vi "Get eq of Time.vi"(6 "Eccentricity":dbl, 9 "Mean Anomaly":dbl, 10 "Geometric Mean Longitude":dbl, 11 "Oblique Correction (deg)":dbl) -> (2 "Eq of Time (min)":dbl, 3 "var y":dbl)   [LabVIEW 2014, in "Solar Calculations.lvlib"]
uses:
  Solar Calculations.lvlib
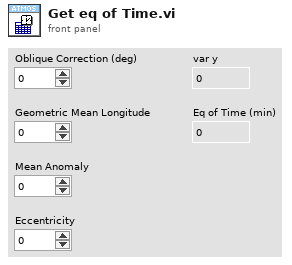
[diagram p1: front panel]
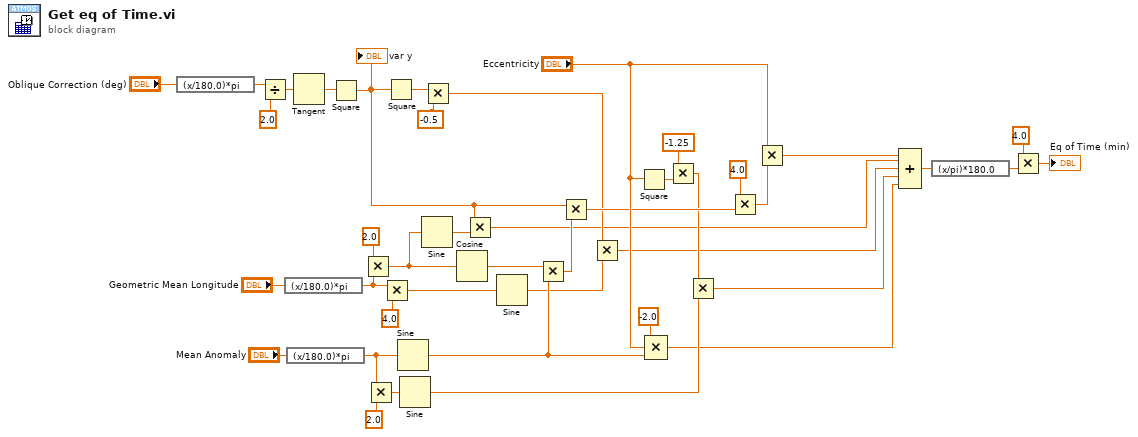
[diagram p0: block diagram]
diagram:
  n1 = expression code="(x/180.0)*pi" ("degrees to radians")("Oblique Correction (deg)") -> (w7:dbl)
  n2 = Divide(x=w7, y=2.0) -> (x/y=w9:dbl)
  n3 = expression code="(x/180.0)*pi" ("degrees to radians")("Geometric Mean Longitude") -> (w36:dbl)
  n4 = expression code="(x/180.0)*pi" ("degrees to radians")("Mean Anomaly") -> (w26:dbl)
  n5 = Tangent(1:w9) -> (0:w10:dbl)
  n6 = Square(x=w10) -> (x^2=w35:dbl)
  "var y" <- w35
  n7 = Multiply(x=2.0, y=w36) -> (x*y=w37:dbl)
  n8 = Multiply(x=w26, y=2.0 ("x")) -> (x*y=w15:dbl)
  n9 = Multiply(x=w36, y=4.0) -> (x*y=w24:dbl)
  n10 = Square(x=w35) -> (x^2=w18:dbl)
  n11 = Sine(x=w26) -> (sin(x)=w32:dbl)
  n12 = Sine(x=w15) -> (sin(x)=w16:dbl)
  n13 = Sine(x=w37) -> (sin(x)=w38:dbl)
  n14 = Multiply(x=w18, y=-0.5) -> (x*y=w20:dbl)
  n15 = Cosine(x=w37) -> (cos(x)=w27:dbl)
  n16 = Multiply(x=w35, y=w38) -> (x*y=w1:dbl)
  n17 = Sine(x=w24) -> (sin(x)=w21:dbl)
  n18 = Multiply(x=w27, y=w32) -> (x*y=w28:dbl)
  n19 = Multiply(x=w35, y=w28) -> (x*y=w29:dbl)
  n20 = Multiply(x=w20, y=w21) -> (x*y=w2:dbl)
  n21 = Square(x="Eccentricity") -> (x^2=w11:dbl)
  n22 = Compound Arithmetic op=MULTIPLY(-2.0 ("value"), "Eccentricity", w32) -> (w3:dbl)
  n23 = Multiply(x=-1.25, y=w11) -> (x*y=w17:dbl)
  n24 = Multiply(x=w17, y=w16) -> (x*y=w4:dbl)
  n25 = Multiply(x=4.0, y=w29) -> (x*y=w31:dbl)
  n26 = Multiply(x="Eccentricity", y=w31) -> (x*y=w5:dbl)
  n27 = Compound Arithmetic op=ADD(w5, w1, w2, w4, w3) -> (w39:dbl)
  n28 = expression code="(x/pi)*180.0" ("radians to degrees")(w39) -> (w40:dbl)
  n29 = Multiply(x=4.0, y=w40) -> (x*y=→"Eq of Time (min)":dbl)
